vi "Reset.vi"(8 "error in (no error)":errorcluster, 11 "Main In":refnum<class "Main.lvclass">) -> (0 "error out":errorcluster, 3 "Main Out":refnum<class "Main.lvclass">)   [LabVIEW 2020, in "Main.lvclass"]
uses:
  Main.lvclass
  Main.lvclass/Main.ctl
  Debugger/Debugger.lvclass
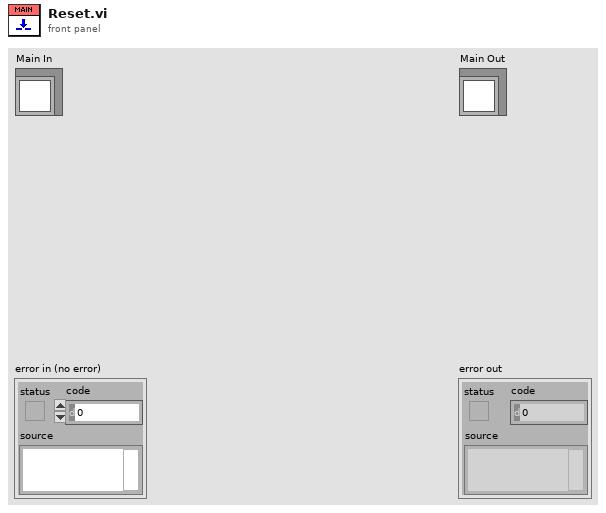
[diagram p1: front panel]
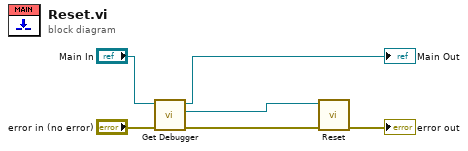
[diagram p0: block diagram]
diagram:
  n1 = call "Get Debugger.vi"("error in (no error)"="error in (no error)", "Main In"="Main In") -> ("error out"=w5:errorcluster, "Debugger.lvclass"=w1:refnum<class "Debugger.lvclass">, "Main Out"=→"Main Out":refnum<class "Main.lvclass">)  [unwired: 7 in]
  n2 = call "Reset.vi"("error in (no error)"=w5, "Debugger in"=w1) -> ("error out"=→"error out":errorcluster)  [unwired: 8 in, 1 out]
